vi "calculate_r2_for_caxis.vi"(8 "Error In":errorcluster, 10 "Expected Angle":dbl, 11 "Xtal Descriptions":T1[](array[typedef])) -> (0 "Error Out":errorcluster, 2 "Theta min":dbl, 3 "Phi min":dbl)   [LabVIEW 2019]
uses:
  xtal_description_for_prediction_cluster_typedef.ctl
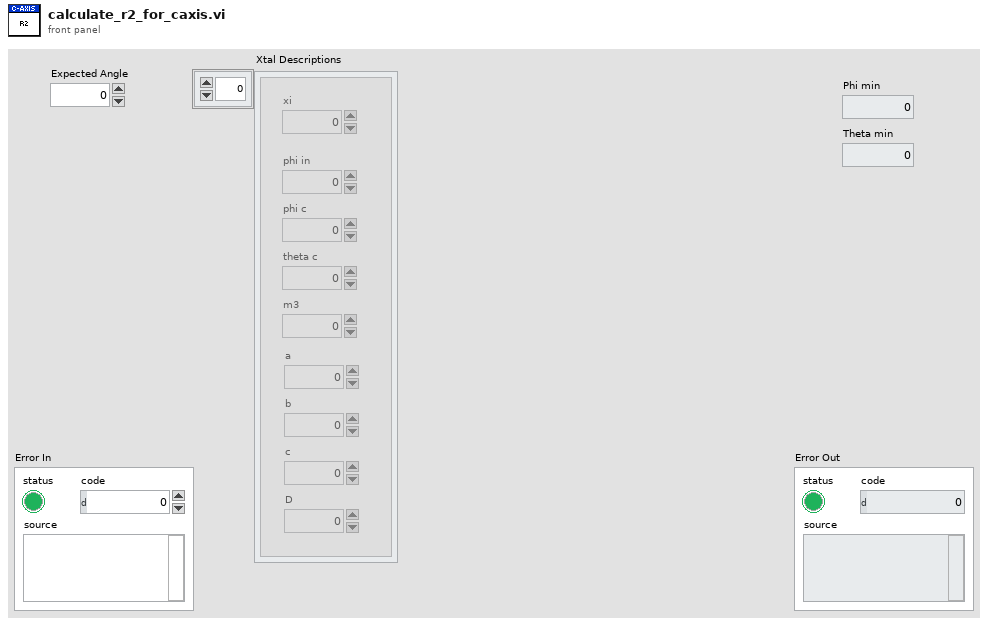
[diagram p1: front panel]
types:
  T1 = typedef "xtal_description_for_prediction_cluster_typedef.ctl" = cluster{"xi":dbl, "phi in":dbl, "phi c":dbl, "theta c":dbl, "m3":dbl, "a":dbl, "b":dbl, "c":dbl, "D":dbl}
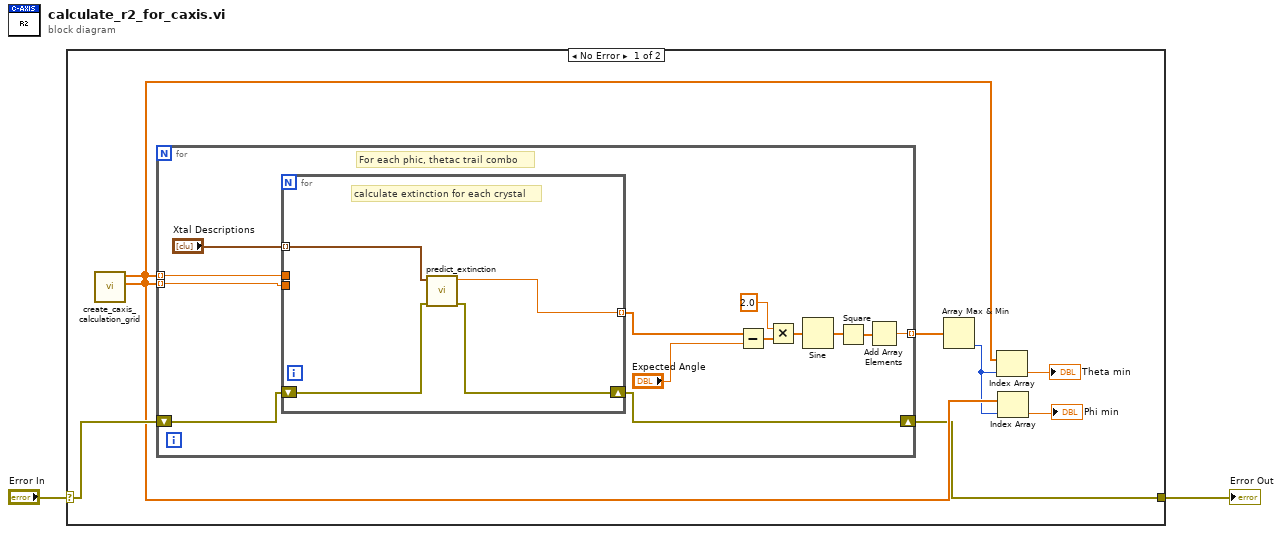
[diagram p0: block diagram]
diagram:
  n1 = case shown="No Error" "Error In" {
    selector: "Error In" -> [w10 w28]
    tunnel: [w3 w28] -> w1
    frame No Error {
      n2 = call "create_caxis_calculation_grid.vi"() -> ("phic"=w7:dbl[], "thetac"=w8:dbl[])  [unwired: 9 in, 1 out]
      n3 = for {
        tunnel: w8 -> [w23] mode=indexing
        tunnel: w7 -> [w22] mode=indexing
        tunnel: [w13] -> w9 mode=indexing
        shift-right: [w11] -> w3
        shift-left: w10 -> [w12]
        # "For each phic, thetac trail combo"
        n4 = for {
          tunnel: w23 -> [_]
          tunnel: w22 -> [_]
          tunnel: [w27] -> w20 mode=indexing
          tunnel: "Xtal Descriptions" -> [w26] mode=indexing
          shift-right: [w25] -> w11
          shift-left: w12 -> [w24]
          # "calculate extinction for each crystal"
          n5 = call "predict_extinction.vi"("Error In"=w24, "Xtal Description"=w26) -> ("Error Out"=w25:errorcluster, "prediction"=w27:dbl)  [unwired: 8 in]
        }
        n6 = Subtract(x=w20, y="Expected Angle") -> (x-y=w18:dbl[])
        n7 = Multiply(x=2.0, y=w18) -> (x*y=w16:dbl[])
        n8 = Sine(x=w16) -> (sin(x)=w15:dbl[])
        n9 = Square(x=w15) -> (x^2=w14:dbl[])
        n10 = Add Array Elements(numeric array=w14) -> (sum=w13:dbl)
      }
      n11 = Array Max & Min(array=w9) -> (min index (indices)=w6:i32)  [unwired: 3 out]
      n12 = Index Array(array=w8, index=w6) -> (element=→"Theta min":dbl)
      n13 = Index Array(array=w7, index=w6) -> (element=→"Phi min":dbl)
    }
    frame Error {
    }
  }
  "Error Out" <- w1
